vi "Configure Acquisition.vi"(8 "error in (no error)":errorcluster, 11 "Scope Base CFG in":refnum<class "Scope Base CFG.lvclass">) -> (0 "error out":errorcluster, 3 "Scope Base CFG out":refnum<class "Scope Base CFG.lvclass">)   [LabVIEW 2023, in "Scope Base CFG.lvclass"]
uses:
  Scope Base CFG.lvclass
  <vilib>/Utility/error.llb/Error Cluster From Error Code.vi
  <vilib>/ErrorRing/Error Ring.xnode
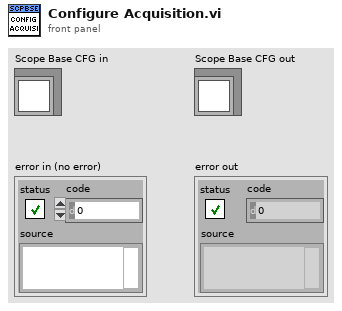
[diagram p1: front panel]
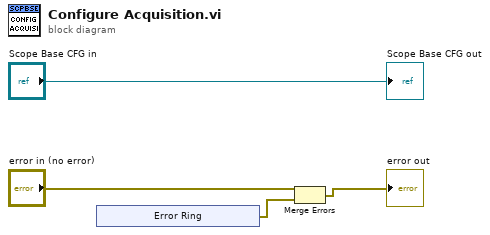
[diagram p0: block diagram]
diagram:
  n1 = xnode "Error Ring"() -> ("error out"=w3:errorcluster)
  n2 = Merge Errors("error in (no error)", w3) -> (→"error out":errorcluster)
  "Scope Base CFG out" <- "Scope Base CFG in"
